vi "Get number of Existing PDOs.vi"(8 "error in (no error)":errorcluster, 11 "Arr Refnum":refnum<vi>) -> (0 "error out":errorcluster, 2 "RX PDOs":u16[](array[numeric]), 3 "TX PDOs":u16[](array[numeric]))   [LabVIEW 2021, in "CANOpen Addon System Explorer.lvlib"]
uses:
  CANOpen Addon System Explorer.lvlib
  control/OD Entry.ctl
  control/Object Type.ctl
  control/Data Type.ctl
  control/Access Type.ctl
  control/OD Cateory.ctl
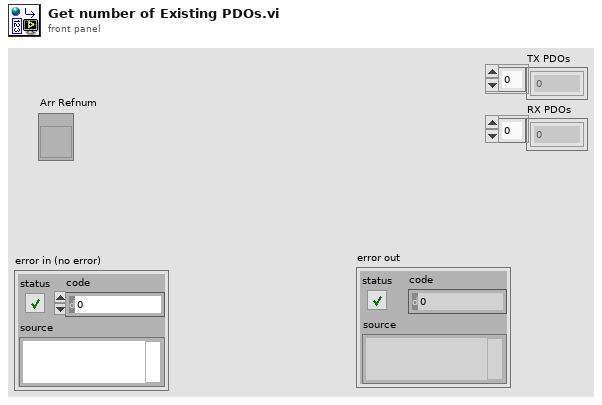
[diagram p1: front panel]
types:
  T1 = typedef "CANOpen Addon System Explorer.lvlib/OD Entry.ctl" = cluster{"index":u16, "sub-index":u8, "Level":u8, "ObjectType":T2, "DataType":T3, "ParameterName":string, "LowLimit":string, "HighLimit":string, "AccessType":T4, "DefaultValue":string, "PDOMapping":bool, "SubNumber":u8, "ObjFlags":u32, "Category":T5}
  T2 = typedef "CANOpen Addon System Explorer.lvlib/Object Type.ctl" = u16
  T3 = typedef "CANOpen Addon System Explorer.lvlib/Data Type.ctl" = u16
  T4 = typedef "CANOpen Addon System Explorer.lvlib/Access Type.ctl" = u16
  T5 = typedef "CANOpen Addon System Explorer.lvlib/OD Cateory.ctl" = enum16{"Mandatory", "Optional", "Manufacturer", ""}
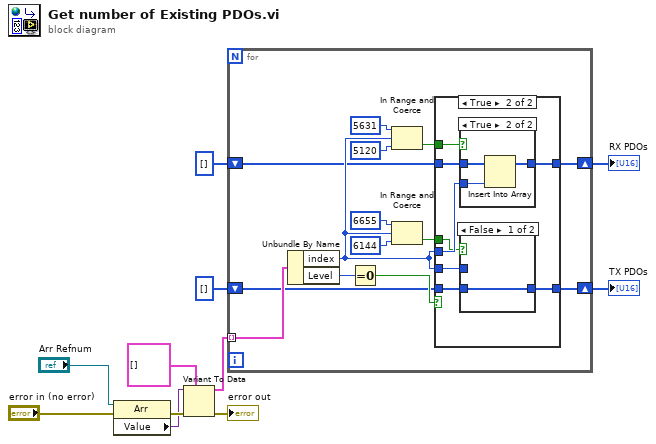
[diagram p0: block diagram]
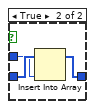
[diagram p3: hidden frame]
diagram:
  n1 = property class="Arr"(reference="Arr Refnum", error in="error in (no error)") -> (error out=w5:errorcluster, "Value"=w4:variant)  [unwired: 1 out]
  n2 = Variant To Data(error in=w5, type=T1[] [], Variant=w4) -> (data=w10:T1[], error out=→"error out":errorcluster)
  n3 = for {
    tunnel: w10 -> [w25] mode=indexing
    shift-right: [w12] -> w1
    shift-left: u16[] [] -> [w15]
    shift-right: [w13] -> w2
    shift-left: u16[] [] -> [w14]
    n4 = Unbundle By Name(w25) -> ("index"=w16:u16, "Level"=w20:u8)
    n5 = Equal To 0?(x=w20) -> (x = 0?=w17:bool)
    n6 = In Range and Coerce(upper limit=u16 5631, x=w16, lower limit=u16 5120) -> (In Range?=w19:bool)  [unwired: 1 out]
    n7 = In Range and Coerce(upper limit=u16 6655, x=w16, lower limit=u16 6144) -> (In Range?=w18:bool)  [unwired: 1 out]
    n8 = case shown="True" w17 {
      tunnel: w19 -> [_ w30]
      tunnel: w18 -> [_ w31]
      tunnel: w16 -> [_ w35]
      tunnel: w16 -> [_ w34]
      tunnel: w15 -> [w27 w33]
      tunnel: w14 -> [w26 w32]
      tunnel: [w26 w29] -> w13
      tunnel: [w27 w28] -> w12
      frame False {
      }
      frame True {
        n9 = case shown="True" w30 {
          tunnel: w35 -> [_ w42]
          tunnel: w33 -> [w40 w43]
          tunnel: [w40 w41] -> w28
          frame False {
          }
          frame True {
            n10 = Insert Into Array(array=w43, new element=w42) -> (w41:u16[])  [unwired: 1 in]
          }
        }
        n11 = case shown="False" w31 {
          tunnel: w34 -> [_ w38]
          tunnel: w32 -> [w36 w39]
          tunnel: [w36 w37] -> w29
          frame False {
          }
          frame True {
            n12 = Insert Into Array(array=w39, new element=w38) -> (w37:u16[])  [unwired: 1 in]
          }
        }
      }
    }
  }
  "TX PDOs" <- w2
  "RX PDOs" <- w1
